vi "CreateObjects.vi"(8 "ErrorIn":errorcluster, 11 "ProgressQueue":refnum<queue>) -> (0 "ErrorOut":errorcluster)   [LabVIEW 2021, in "Application.lvclass"]
doc: "Calls the Create method from each of the objects in the pool if these objects supports the ICreateDestroy interface. If they don't support it the object is skipped"
uses:
  Application.lvclass
  Interface_Object_ICreateDestroy/ICreateDestroy/ICreateDestroy.lvclass
  Interface_TAF_ITAFObject/ITAFObject/ITAFObject.lvclass
  5c5df808-c013-4a6b-85e3-bbe17662ba10.vi
  18a8f3d7-0e6d-4485-acbc-c4a53fef0119.vi
  <vilib>/TriekselSoft/TracerLibrary/TracerLibrary/Tracer/protected/SendMessage.vi
  <vilib>/TriekselSoft/TracerLibrary/TracerLibrary/Tracer/protected/Timestamp.vi
  18a8f3d7-0e6d-4485-acbc-c4a53fef0119.vi/f75db090-0877-4668-94fb-75c2140b1617.vi
  <vilib>/TriekselSoft/TracerLibrary/TracerLibrary/Tracer/Tracer_Level-Debug.vi
  <vilib>/TriekselSoft/TracerLibrary/TracerLibrary/Tracer/protected/Tracer_ClassAttributes.vi
  <vilib>/JDP Science/JSONtext/Variant to JSON Text.vi
  <vilib>/JDP Science/JSONtext/LVClass Serializer/JSONtext LVClass Serializer.lvclass
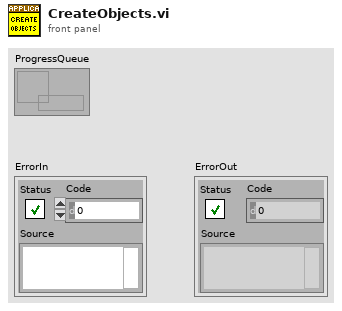
[diagram p1: front panel]
types:
  T1 = typedef "Application.lvclass/ObjectAttributes.ctl" = cluster{"Objects":variant, "BasePath":path, "Application":refnum<class "Application.lvclass">}
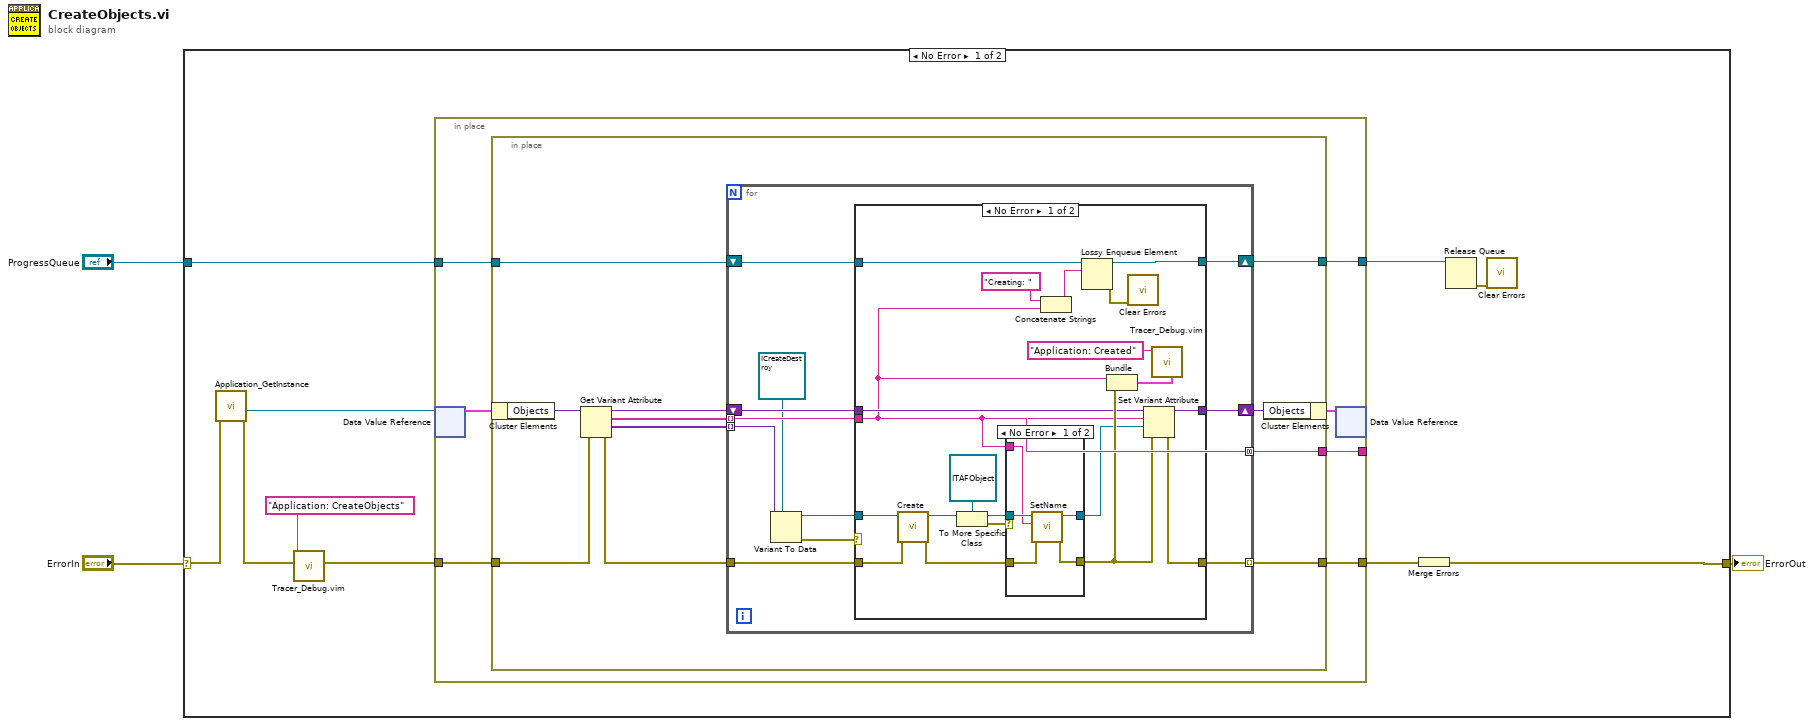
[diagram p0: block diagram]
diagram:
  n1 = case shown="No Error" "ErrorIn" {
    selector: "ErrorIn" -> [w12 w73]
    tunnel: [w9 w73] -> w2
    tunnel: "ProgressQueue" -> [w7 _]
    frame No Error {
      n2 = call "Application_GetInstance.vi"("ErrorIn"=w12) -> ("ErrorOut"=w11:errorcluster, "DVRRefOut"=w5:refnum<data-value>)  [unwired: 6 in, 3 out]
      n3 = call "Tracer_Debug.vim"("Error In"=w11, "Text"="Application: CreateObjects") -> ("Error Out"=w10:errorcluster)  [unwired: 9 in]
      n4 = in-place {
        in-place-border: w10 -> [w20]
        in-place-border: [w19] -> _
        in-place-border: w7 -> [w18]
        in-place-border: [w17] -> w6
        in-place-border: [w14] -> w4
        n5 = in-place-dvr #1(w5) -> (w16:T1)  [unwired: 1 out]
        n6 = in-place {
          in-place-border: w20 -> [w30]
          in-place-border: [w29] -> w19
          in-place-border: w18 -> [w28]
          in-place-border: [w27] -> w17
          in-place-border: [w21] -> w14
          n7 = in-place-cluster #2(w16) -> ("Objects"=w25:variant)
          n8 = Get Variant Attribute(Variant=w25, error in=w30) -> (duplicate Variant=w24:variant, names=w22:string[], values=w23:variant[], error out=w31:errorcluster)  [unwired: 2 in]
          n9 = for {
            tunnel: w31 -> [w42]
            tunnel: [w35] -> w29 mode=concatenating
            shift-right: [w38] -> w27
            shift-left: w28 -> [w39]
            shift-right: [w36] -> w26
            shift-left: w24 -> [w37]
            tunnel: w23 -> [w34] mode=indexing
            tunnel: w22 -> [w35] mode=indexing
            tunnel: [w40] -> w21 mode=indexing
            n10 = Variant To Data(type=refnum<class "ICreateDestroy.lvclass"> refnum ("ICreateDestroy"), Variant=w34) -> (data=w32:refnum<class "ICreateDestroy.lvclass">, error out=w41:errorcluster)  [unwired: 1 in]
            n11 = case shown="No Error" w41 {
              tunnel: w39 -> [w56 w71]
              tunnel: [w55 w71] -> w38
              tunnel: w37 -> [w54 w70]
              tunnel: [w53 w70] -> w36
              tunnel: w35 -> [w44 _]
              tunnel: w42 -> [w61 w72]
              tunnel: w32 -> [w50 _]
              tunnel: [w60 w72] -> w40
              frame No Error {
                n12 = call-dynamic "Create.vi"("ErrorIn"=w61, "ObjectIn"=w50) -> ("ErrorOut"=w57:errorcluster, "ObjectOut"=w47:refnum<class "ICreateDestroy.lvclass">)  [unwired: 8 in]
                n13 = To More Specific Class(target class=refnum<class "ITAFObject.lvclass"> refnum ("object in"), reference=w47) -> (specific class reference=w45:refnum<class "ITAFObject.lvclass">, error out=w59:errorcluster)  [unwired: 1 in]
                n14 = case shown="No Error" w59 {
                  tunnel: w57 -> [w67 w69]
                  tunnel: [w66 w69] -> w58
                  tunnel: w45 -> [w65 w68]
                  tunnel: w44 -> [w64 _]
                  tunnel: [w63 w68] -> w43
                  frame No Error {
                    n15 = call-dynamic "SetName.vi"("ErrorIn"=w67, "Name"=w64, "ObjectIn"=w65) -> ("ErrorOut"=w66:errorcluster, "ObjectOut"=w63:refnum<class "ITAFObject.lvclass">)  [unwired: 7 in]
                  }
                  frame Error {
                  }
                }
                n16 = Concatenate Strings("Creating: " ("string"), w44) -> (w52:string)
                n17 = Lossy Enqueue Element(queue=w56, element=w52) -> (queue out=w55:refnum<queue>, error out=w62:errorcluster)  [unwired: 1 in, 2 out]
                n18 = Bundle(w44, "ErrorOut"=w58) -> (w48:cluster{string, "ErrorOut":errorcluster})  [unwired: 1 in]
                n19 = call <vilib>:"Clear Errors.vi"("error in (no error)"=w62) -> ()  [unwired: 5 in, 2 out]
                n20 = Set Variant Attribute(Variant=w54, name=w44, value=w43, error in=w58) -> (Variant out=w53:variant, error out=w60:errorcluster)  [unwired: 1 out]
                n21 = call "Tracer_Debug.vim"("Data"=w48, "Text"="Application: Created") -> ()  [unwired: 9 in, 1 out]
              }
              frame Error {
              }
            }
          }
          n22 = in-place-cluster #2("Objects"=w26) -> (w15:T1)
        }
        n23 = in-place-dvr #1(w15) -> ()  [unwired: 2 out]
      }
      n24 = Merge Errors(w4) -> (w9:errorcluster)
      n25 = Release Queue(queue=w6) -> (error out=w13:errorcluster)  [unwired: 2 in, 2 out]
      n26 = call <vilib>:"Clear Errors.vi"("error in (no error)"=w13) -> ()  [unwired: 5 in, 2 out]
    }
    frame Error {
    }
  }
  "ErrorOut" <- w2
